vi "RSNRPZ Fetch Buffer Data Aux.vi"(7 "Buffer Size (0)":i32, 8 "error in (no error)":errorcluster, 9 "Maximum Time (5000 ms)":i32=5000, 10 "Channel (1)":i32=1, 11 "VISA session":refnum<visa-resource-name> caption="VISA resource name") -> (0 "error out":errorcluster, 1 "Aux 1 Array":dbl[](array[numeric]) format="%^.3e", 2 "Measurement Array":dbl[](array[numeric]) format="%^.3e", 3 "dup VISA session":refnum<visa-resource-name> caption="VISA resource name", 4 "Aux 2 Array":dbl[](array[numeric]) format="%^.3e", 5 "Read Count":i32)   [LabVIEW 2010]
doc: "This VI returns the buffer measurement the sensor acquires for the channel you specify. The measurement is from an acquisition that you previously initiated. \n\nYou use the rsnrpz_chan_initiate VI to start an acquisition on the channels that you specify. You use the rsnrpz_chan_isMeasurementComplete VI to determine when the acquisition is complete.\n\nYou can call the rsnrpz_meas_readBufferMeasurement VI instead of the rsnrpz_chan_initiate VI. The rsnrpz_meass_readBufferMeasurement VI starts an acquisition, waits for the acquisition to complete, and returns the measurement for the channel you specify.\n\nNote:\n\n1) If the acquisition has not be initialized or measurement is still in progress and value is not available, VI returns an error( RSNRPZ_ERROR_MEAS_NOT_AVAILABLE ).\n\n2) If SENSE:AUX is set to None, this VI returns error."
uses:
  rsnrpz_32.dll
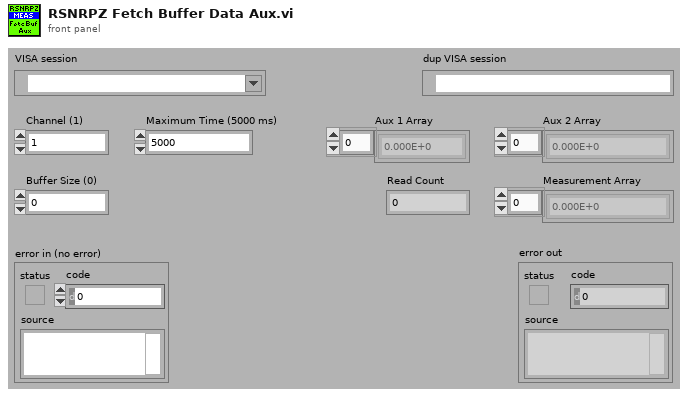
[diagram p1: front panel]
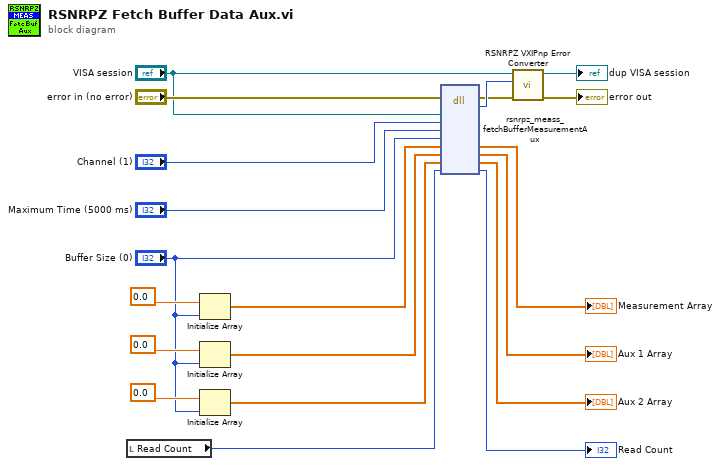
[diagram p0: block diagram]
diagram:
  n1 = local read "Read Count"() -> (w8:i32)
  n2 = Initialize Array(0.0, "Buffer Size (0)") -> (w14:dbl[])
  n3 = Initialize Array(0.0, "Buffer Size (0)") -> (w12:dbl[])
  n4 = Initialize Array(0.0, "Buffer Size (0)") -> (w10:dbl[])
  n5 = dll-call lib="rsnrpz_32.dll" fn="rsnrpz_meass_fetchBufferMeasurementAux"(error in="error in (no error)", "Instrument Handle"="VISA session", "Channel"="Channel (1)", "Maximum Time (ms)"="Maximum Time (5000 ms)", "Buffer Size"="Buffer Size (0)", "Measurement Array"=w14, "Aux 1 Array"=w12, "Aux 2 Array"=w10, "Read Count"=w8) -> (error out=w5:errorcluster, "Status"=w17:i32, "Measurement Array"=→"Measurement Array":dbl[], "Aux 1 Array"=→"Aux 1 Array":dbl[], "Aux 2 Array"=→"Aux 2 Array":dbl[], "Read Count"=→"Read Count":i32)  [unwired: 6 in, 1 out]
  n6 = call <instrlib>:"RSNRPZ VXIPnp Error Converter.vi"("error in"=w5, "VXIPnp error code"=w17, "VISA session"="VISA session") -> ("error out"=→"error out":errorcluster, "dup VISA session"=→"dup VISA session":refnum<visa-resource-name>)  [unwired: 7 in]
